vi "start com.vi"(2 "COM DATA":T1) -> (0 "ONLINE OUT":T2={"connection ID"=refnum, "Time Out"=0, "error out"={"status"=TRUE, "code"=0, "source"=""}})   [LabVIEW 2010]
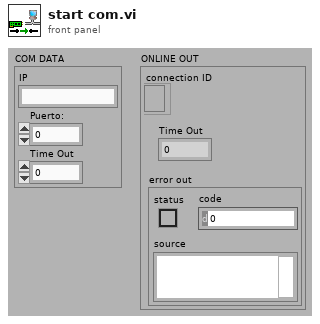
[diagram p1: front panel]
types:
  T1 = cluster{"IP ":string, "Puerto:":u16, "Time Out":u16}
  T2 = cluster{"connection ID":refnum<k5>, "Time Out":u16, "error out":errorcluster}
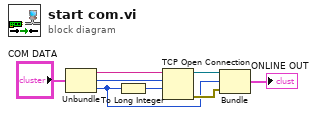
[diagram p0: block diagram]
diagram:
  n1 = Unbundle("COM DATA") -> ("IP"=w7:string, "Puerto:"=w6:u16, "Time Out"=w1:u16)
  n2 = To Long Integer(number=w1) -> (32bit integer=w2:i32)
  n3 = TCP Open Connection(address=w7, remote port or service name=w6, timeout ms (60000)=w2) -> (connection ID=w5:refnum<k5>, error out=w3:errorcluster)  [unwired: 2 in]
  n4 = Bundle("connection ID"=w5, "Time Out"=w1, "error out"=w3) -> (→"ONLINE OUT":T2)  [unwired: 1 in]
